vi "SDSU_AttHandling.vi"(8 "error IO":errorcluster, 10 "arguments":string, 11 "refnum":i32) -> (0 "err out":errorcluster, 2 "response":string, 3 "refnum out":i32)   [LabVIEW 2016]
uses:
  DBSHAND/private/vis/DatabaseHand_Element_Get(string).vi
  DBSHAND/private/vis/DatabaseHand_Element_Set(string).vi
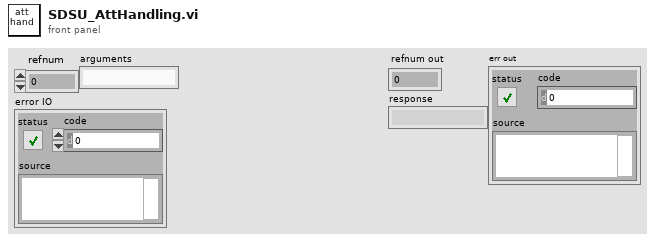
[diagram p1: front panel]
types:
  T1 = typedef "DatabaseHand_RefNum.ctl" = refnum<vi>
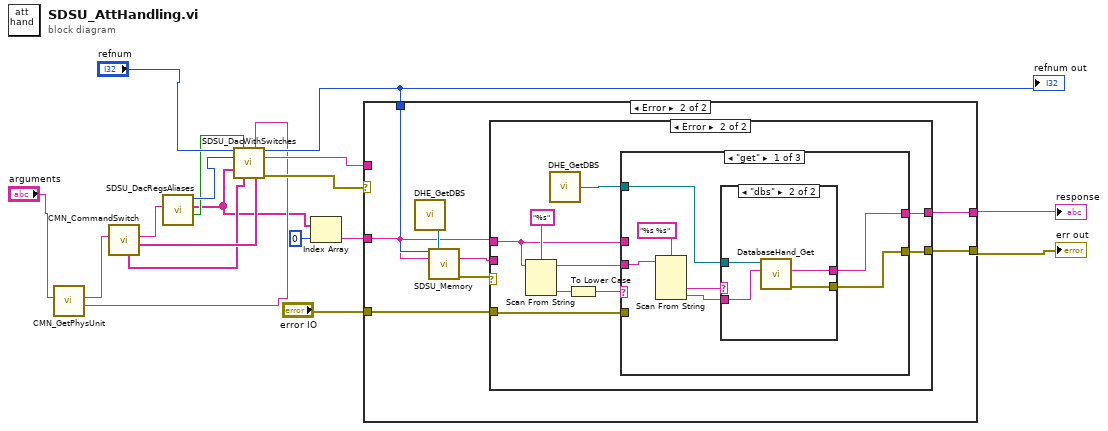
[diagram p0: block diagram]
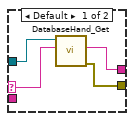
[diagram p4: hidden frame]
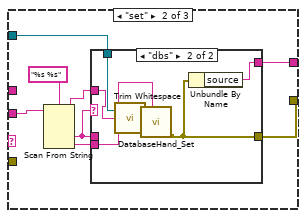
[diagram p5: hidden frame]
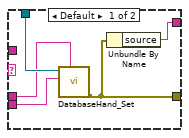
[diagram p6: hidden frame]
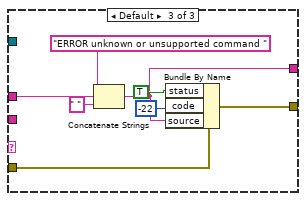
[diagram p7: hidden frame]
diagram:
  n1 = call "CMN_GetPhysUnit.vi"("command in"="arguments") -> ("unit"=w5:string, "command out"=w15:string)  [unwired: 9 out]
  n2 = call "CMN_CommandSwitch.vi"("command in"=w15) -> ("swhitches"=w9:string[], "command out"=w13:string, "arguments"=w8:string[])  [unwired: 1 in, 7 out]
  n3 = call "SDSU_DacRegsAliases.vi"("cmd in"=w13) -> ("register?"=w6:bool, "cmds out"=w3:string[], "first reg"=w7:i32)  [unwired: 7 in, 1 out]
  n4 = call "SDSU_DacWithSwitches.vi"("refnum"="refnum", "register"=w6, "unit"=w5, "first reg"=w7, "cmds"=w3, "sw args"=w8, "swhitches"=w9) -> ("refnum out"=w18:i32, "response"=w11:string, "error out"=w12:errorcluster)  [unwired: 6 in]
  "refnum out" <- w18
  n5 = Index Array(array=w3, index=0) -> (element=w1:string)
  n6 = case shown="Error" w12 {
    selector: w12 -> [w19 _]
    tunnel: "error IO" -> [_ w28]
    tunnel: [w19 w27] -> w16
    tunnel: [w20 w26] -> w4
    tunnel: w11 -> [w20 _]
    tunnel: w18 -> [_ w24]
    tunnel: w1 -> [_ w21]
    frame No Error {
    }
    frame Error {
      n7 = call "DHE_GetDBS.vi"() -> ("DHE_DBSRef"=w25:T1)  [unwired: 9 out]
      n8 = call "SDSU_Memory.vi"("refnum"=w24, "Database RefNum in"=w25, "Command In"=w21) -> ("message"=w22:string, "error out"=w23:errorcluster)  [unwired: 2 in, 9 out]
      n9 = case shown="Error" w23 {
        selector: w23 -> [w29 _]
        tunnel: w28 -> [_ w39]
        tunnel: [w29 w38] -> w27
        tunnel: w21 -> [_ w31]
        tunnel: [w30 w37] -> w26
        tunnel: w22 -> [w30 _]
        frame No Error {
        }
        frame Error {
          n10 = Scan From String(format string="%s", input string=w31) -> (remaining string=w32:string, output 1=w35:string)  [unwired: 3 in, 2 out]
          n11 = call "DHE_GetDBS.vi"() -> ("DHE_DBSRef"=w33:T1)  [unwired: 9 out]
          n12 = To Lower Case(string=w35) -> (all lower case string=w34:string)
          n13 = case shown="\"get\"" w34 {
            tunnel: w39 -> [_ _ w81]
            tunnel: [w42 w58 w79] -> w38
            tunnel: w31 -> [_ _ w76]
            tunnel: [w43 w57 w74] -> w37
            tunnel: w33 -> [w46 w60 _]
            tunnel: w32 -> [w45 w62 _]
            frame "get" {
              n14 = Scan From String(format string="%s %s", input string=w45) -> (output 1=w41:string, output 2=w40:string)  [unwired: 4 in, 3 out]
              n15 = case shown="\"dbs\"" w41 {
                selector: w41 -> [w49 _]
                tunnel: w46 -> [w50 w54]
                tunnel: [w48 w53] -> w43
                tunnel: [w47 w52] -> w42
                tunnel: w40 -> [_ w51]
                frame Default {
                  n16 = call-poly "DatabaseHand_Get.vi"("name"=w49, "Database RefNum in"=w50) -> ("error out"=w47:errorcluster, "value"=w48:string)  [unwired: 3 in, 5 out]
                }
                frame "dbs" {
                  n17 = call-poly "DatabaseHand_Get.vi"("name"=w51, "Database RefNum in"=w54) -> ("error out"=w52:errorcluster, "value"=w53:string)  [unwired: 3 in, 5 out]
                }
              }
            }
            frame "set" {
              n18 = Scan From String(format string="%s %s", input string=w62) -> (remaining string=w55:string, output 1=w56:string, output 2=w59:string)  [unwired: 4 in, 2 out]
              n19 = case shown="\"dbs\"" w56 {
                tunnel: w60 -> [w67 w73]
                tunnel: w56 -> [w66 _]
                tunnel: w59 -> [w65 w70]
                tunnel: [w64 w72] -> w58
                tunnel: [w63 w71] -> w57
                tunnel: w55 -> [_ w69]
                frame Default {
                  n20 = call-poly "DatabaseHand_Set.vi"("name"=w66, "value"=w65, "Database RefNum in"=w67) -> ("error out"=w64:errorcluster)  [unwired: 7 in, 1 out]
                  n21 = Unbundle By Name(w64) -> ("source"=w63:string)
                }
                frame "dbs" {
                  n22 = call <vilib>:"Trim Whitespace.vi"("string"=w69) -> ("trimmed string"=w68:string)  [unwired: 1 in]
                  n23 = call-poly "DatabaseHand_Set.vi"("name"=w70, "value"=w68, "Database RefNum in"=w73) -> ("error out"=w72:errorcluster)  [unwired: 7 in, 1 out]
                  n24 = Unbundle By Name(w72) -> ("source"=w71:string)
                }
              }
            }
            frame Default {
              n25 = Concatenate Strings("ERROR unknown or unsupported command " ("source"), w76, " " ("string")) -> (w74:string)
              n26 = Bundle By Name(cluster=w81, "status"=TRUE, "code"=-22, "source"=w74) -> (w79:errorcluster)
            }
          }
        }
      }
    }
  }
  "response" <- w4
  "err out" <- w16
